vi "After Launch Init Core.vi"(8 "error in (no error)":errorcluster, 10 "DelayInitialization?":bool, 11 "BNT_DAQmx-MCSV in":refnum<class "BNT_DAQmx-MCSV.lvclass">) -> (0 "error out":errorcluster, 3 "BNT_DAQmx-MCSV out":refnum<class "BNT_DAQmx-MCSV.lvclass">)   [LabVIEW 2019, in "BNT_DAQmx.lvlib" / "BNT_DAQmx-MCSV.lvclass"]
doc: "Use <b>Pre Launch init.vi</b> method for sanity checks that are supposed to prevent the actor from launching if they fail. Use <B>this</B> method instead to initialize this actor when it has been activated. A corresponding high priority message will become dispatched before the <B>Actor Core.vi</b> is called.\n\n<b>Derived classed should call the parent methode first</b> and their own initialization code after.\n\nRefer also to the ongoing discussion at https://decibel.ni.com/content/message/57394#57394."
uses:
  BNT_DAQmx-MCSV.lvclass
  CSPP_Core/Classes/CSPP_ProcessVariables/CSPP_ProcessVariables.lvlib
  CSPP_Core/Actors/CSPP_DeviceActor/CSPP_DeviceActor.lvclass
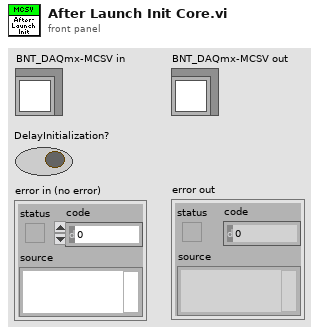
[diagram p1: front panel]
types:
  T1 = cluster{"Write Access":enum8{"Allowed", "Required", "None"}, "Read Access":enum8{"Allowed", "Required", "None"}}
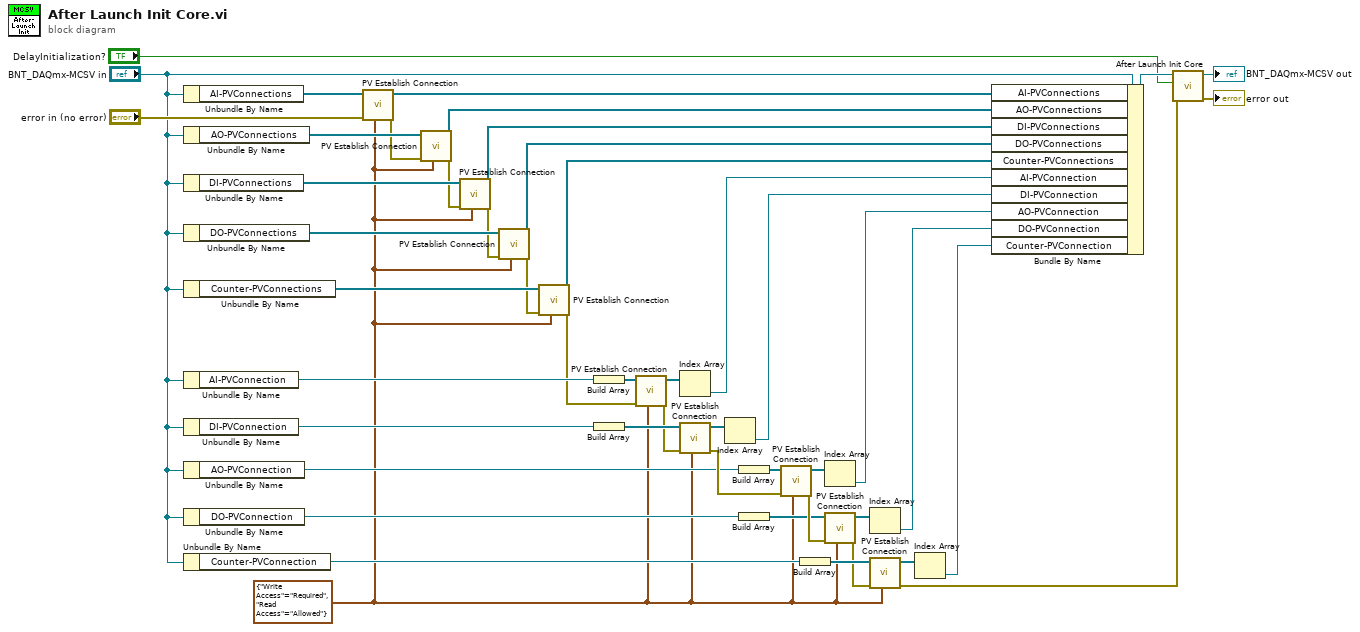
[diagram p0: block diagram]
diagram:
  w5 = T1 {"Write Access"=enum."Required", "Read Access"=enum."Allowed"} ("Access")
  n1 = Unbundle By Name("BNT_DAQmx-MCSV in") -> ("AI-PVConnections"=w42:refnum<class "PVConnection.lvclass">[])
  n2 = Unbundle By Name("BNT_DAQmx-MCSV in") -> ("AO-PVConnections"=w44:refnum<class "PVConnection.lvclass">[])
  n3 = Unbundle By Name("BNT_DAQmx-MCSV in") -> ("DI-PVConnections"=w38:refnum<class "PVConnection.lvclass">[])
  n4 = Unbundle By Name("BNT_DAQmx-MCSV in") -> ("DO-PVConnections"=w37:refnum<class "PVConnection.lvclass">[])
  n5 = Unbundle By Name("BNT_DAQmx-MCSV in") -> ("Counter-PVConnections"=w6:refnum<class "PVConnection.lvclass">[])
  n6 = Unbundle By Name("BNT_DAQmx-MCSV in") -> ("AI-PVConnection"=w32:refnum<class "PVConnection.lvclass">)
  n7 = Unbundle By Name("BNT_DAQmx-MCSV in") -> ("DI-PVConnection"=w16:refnum<class "PVConnection.lvclass">)
  n8 = Unbundle By Name("BNT_DAQmx-MCSV in") -> ("AO-PVConnection"=w15:refnum<class "PVConnection.lvclass">)
  n9 = Unbundle By Name("BNT_DAQmx-MCSV in") -> ("DO-PVConnection"=w14:refnum<class "PVConnection.lvclass">)
  n10 = Unbundle By Name("BNT_DAQmx-MCSV in") -> ("Counter-PVConnection"=w11:refnum<class "PVConnection.lvclass">)
  n11 = call "PV Establish Connection.vi"("Access (R/W allowed)"=w5, "Error In"="error in (no error)", "PVConnections in"=w42) -> ("Error Out"=w39:errorcluster, "PVConnections out"=w41:refnum<class "PVConnection.lvclass">[])  [unwired: 7 in]
  n12 = call "PV Establish Connection.vi"("Access (R/W allowed)"=w5, "Error In"=w39, "PVConnections in"=w44) -> ("Error Out"=w35:errorcluster, "PVConnections out"=w43:refnum<class "PVConnection.lvclass">[])  [unwired: 7 in]
  n13 = call "PV Establish Connection.vi"("Access (R/W allowed)"=w5, "Error In"=w35, "PVConnections in"=w38) -> ("Error Out"=w36:errorcluster, "PVConnections out"=w34:refnum<class "PVConnection.lvclass">[])  [unwired: 7 in]
  n14 = call "PV Establish Connection.vi"("Access (R/W allowed)"=w5, "Error In"=w36, "PVConnections in"=w37) -> ("Error Out"=w4:errorcluster, "PVConnections out"=w33:refnum<class "PVConnection.lvclass">[])  [unwired: 7 in]
  n15 = call "PV Establish Connection.vi"("Access (R/W allowed)"=w5, "Error In"=w4, "PVConnections in"=w6) -> ("Error Out"=w3:errorcluster, "PVConnections out"=w2:refnum<class "PVConnection.lvclass">[])  [unwired: 7 in]
  n16 = Build Array(w32) -> (w31:refnum<class "PVConnection.lvclass">[])
  n17 = Build Array(w16) -> (w27:refnum<class "PVConnection.lvclass">[])
  n18 = call "PV Establish Connection.vi"("Access (R/W allowed)"=w5, "Error In"=w3, "PVConnections in"=w31) -> ("Error Out"=w26:errorcluster, "PVConnections out"=w30:refnum<class "PVConnection.lvclass">[])  [unwired: 7 in]
  n19 = Index Array(array=w30) -> (element=w29:refnum<class "PVConnection.lvclass">)  [unwired: 1 in]
  n20 = call "PV Establish Connection.vi"("Access (R/W allowed)"=w5, "Error In"=w26, "PVConnections in"=w27) -> ("Error Out"=w19:errorcluster, "PVConnections out"=w28:refnum<class "PVConnection.lvclass">[])  [unwired: 7 in]
  n21 = Index Array(array=w28) -> (element=w25:refnum<class "PVConnection.lvclass">)  [unwired: 1 in]
  n22 = Build Array(w15) -> (w20:refnum<class "PVConnection.lvclass">[])
  n23 = Build Array(w14) -> (w23:refnum<class "PVConnection.lvclass">[])
  n24 = call "PV Establish Connection.vi"("Access (R/W allowed)"=w5, "Error In"=w19, "PVConnections in"=w20) -> ("Error Out"=w24:errorcluster, "PVConnections out"=w21:refnum<class "PVConnection.lvclass">[])  [unwired: 7 in]
  n25 = Build Array(w11) -> (w12:refnum<class "PVConnection.lvclass">[])
  n26 = Index Array(array=w21) -> (element=w18:refnum<class "PVConnection.lvclass">)  [unwired: 1 in]
  n27 = call "PV Establish Connection.vi"("Access (R/W allowed)"=w5, "Error In"=w24, "PVConnections in"=w23) -> ("Error Out"=w10:errorcluster, "PVConnections out"=w22:refnum<class "PVConnection.lvclass">[])  [unwired: 7 in]
  n28 = Index Array(array=w22) -> (element=w17:refnum<class "PVConnection.lvclass">)  [unwired: 1 in]
  n29 = call "PV Establish Connection.vi"("Access (R/W allowed)"=w5, "Error In"=w10, "PVConnections in"=w12) -> ("Error Out"=w9:errorcluster, "PVConnections out"=w13:refnum<class "PVConnection.lvclass">[])  [unwired: 7 in]
  n30 = Index Array(array=w13) -> (element=w8:refnum<class "PVConnection.lvclass">)  [unwired: 1 in]
  n31 = Bundle By Name(cluster="BNT_DAQmx-MCSV in", "AI-PVConnections"=w41, "AO-PVConnections"=w43, "DI-PVConnections"=w34, "DO-PVConnections"=w33, "Counter-PVConnections"=w2, "AI-PVConnection"=w29, "DI-PVConnection"=w25, "AO-PVConnection"=w18, "DO-PVConnection"=w17, "Counter-PVConnection"=w8) -> (w47:refnum<class "BNT_DAQmx-MCSV.lvclass">)
  n32 = call-parent "After Launch Init Core.vi"("error in (no error)"=w9, "DelayInitialization?"="DelayInitialization?", "CSPP_DeviceActor in"=w47) -> ("error out"=→"error out":errorcluster, "CSPP_DeviceActor out"=→"BNT_DAQmx-MCSV out":refnum<class "BNT_DAQmx-MCSV.lvclass">)  [unwired: 7 in]
